vi "WORD report.vi"(7 "Report state":T1=enum."Close report", 8 "error in":errorcluster, 10 "Data in":variant) -> (0 "error out":errorcluster, 2 "Data out":variant)   [LabVIEW 2015, in "Report.lvlib"]
uses:
  Report.lvlib
  <vilib>/Utility/NIReport.llb/NI_report.lvclass
  <vilib>/Utility/NIReport.llb/Append Report Text (str wrap).vi
  <vilib>/Utility/NIReport.llb/NI_ReportGenerationCore.lvlib
  TypeDefs/Report data.ctl
  TypeDefs/Report state.ctl
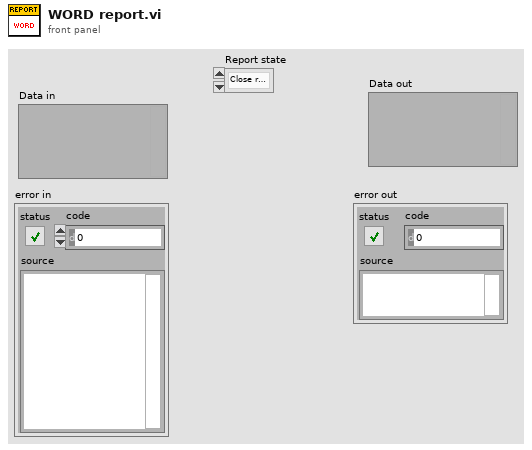
[diagram p1: front panel]
types:
  T1 = typedef "Report.lvlib/Report state.ctl" = enum16{"Create report", "Save data", "Save report", "Available printers", "Print report", "Close report"}
  T2 = enum16{"maximized", "minimized", "normal", "no change"}
  T3 = enum16{"Standard Report", "HTML", "Word", "Excel"}
  T4 = typedef "Report.lvlib/Report data.ctl" = cluster{"report ID":refnum<class "NI_report.lvclass">, "error":errorcluster}
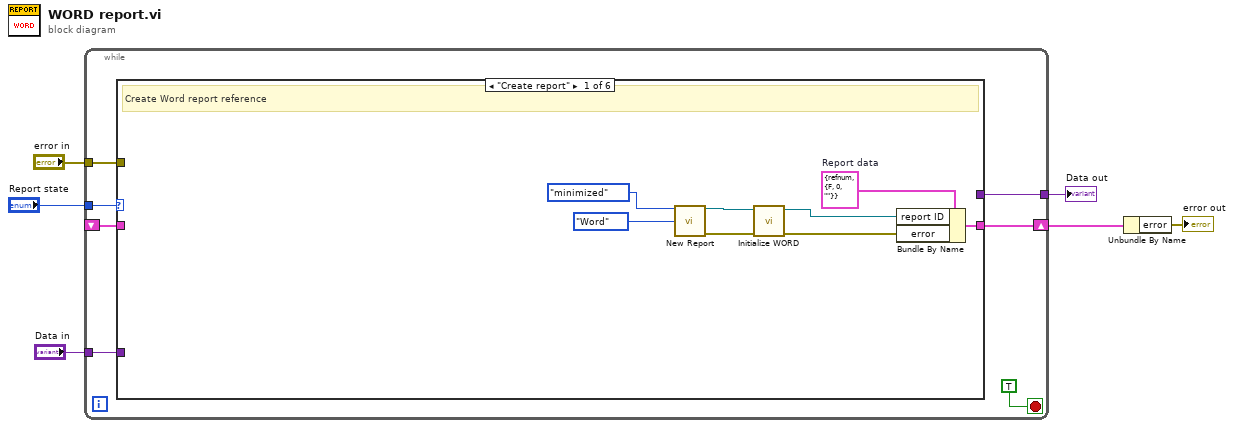
[diagram p0: block diagram]
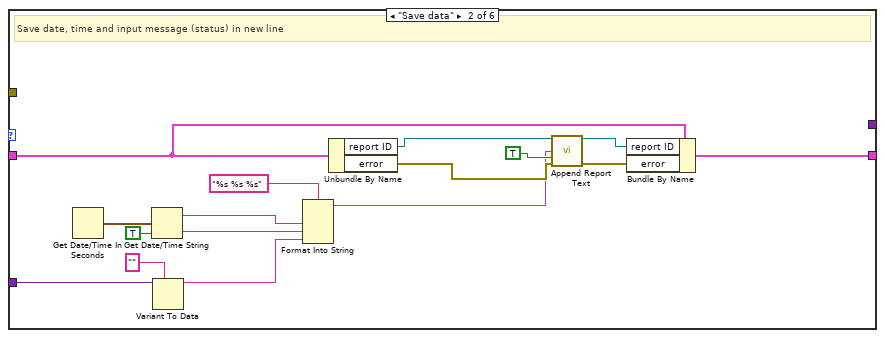
[diagram p2: hidden frame]
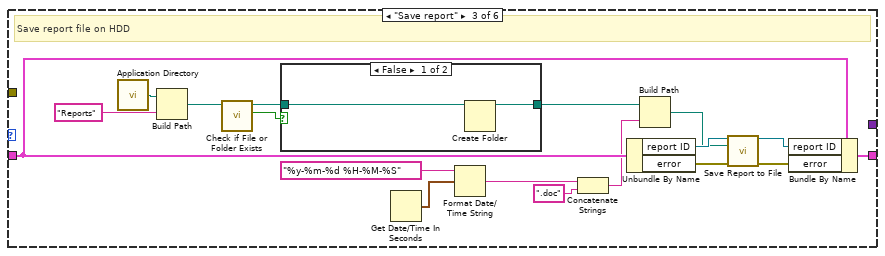
[diagram p3: hidden frame]
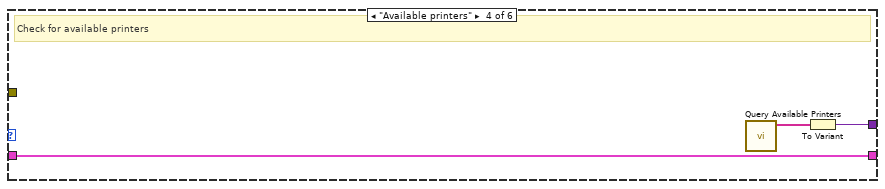
[diagram p5: hidden frame]
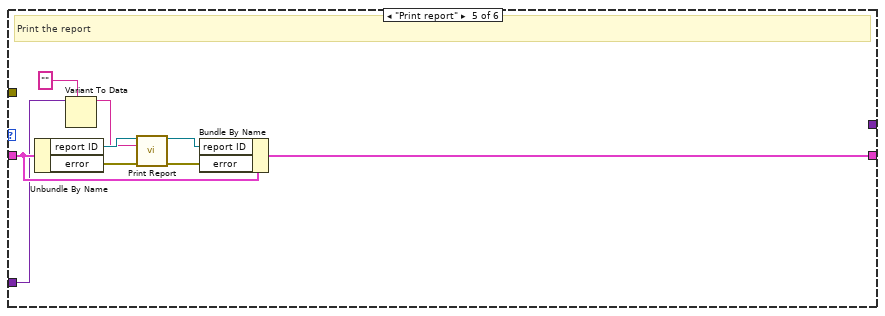
[diagram p6: hidden frame]
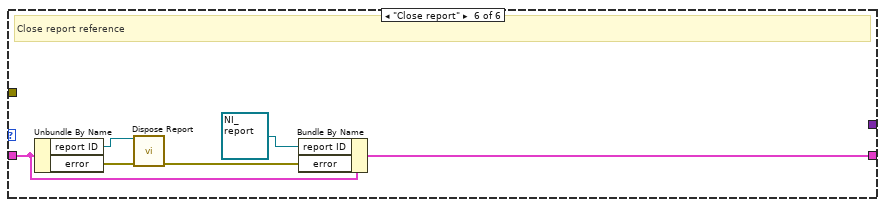
[diagram p7: hidden frame]
diagram:
  n1 = while {
    tunnel: "Report state" -> [w9]
    shift-right: [w11] -> w3
    shift-left: _ -> [w12]
    tunnel: "Data in" -> [w10]
    tunnel: "error in" -> [w8]
    tunnel: [w7] -> w1
    stop <- TRUE stop-if-true
    n2 = case shown="\"Create report\"" w9 {
      tunnel: w12 -> [_ w35 w55 w59 w68 w75]
      tunnel: [w21 w32 w54 w59 w67 w76] -> w11
      tunnel: w10 -> [_ w31 _ _ w64 _]
      tunnel: w8 -> [_ _ _ _ _ _]
      tunnel: [_ _ _ w60 _ _] -> w7
      frame "Create report" {
        w14 = T4 {"report ID"=refnum, "error"={"status"=FALSE, "code"=0, "source"=""}}  # Report data
        # "Create Word report reference"
        n3 = call <vilib>:"New Report.vi"("window state (normal)"=T2."minimized", "report type"=T3."Word") -> ("report out"=w18:refnum<class "NI_report.lvclass">, "error out"=w17:errorcluster)  [unwired: 12 in]
        n4 = call "Initialize WORD.vi"("error in (no error)"=w17, "NI_report in"=w18) -> ("error out"=w15:errorcluster, "NI_report out"=w16:refnum<class "NI_report.lvclass">)  [unwired: 8 in]
        n5 = Bundle By Name(cluster=w14, "report ID"=w16, "error"=w15) -> (w21:T4)
      }
      frame "Save data" {
        # "Save date, time and input message (status) in new line"
        n6 = Get Date/Time In Seconds() -> (seconds since 1Jan1904=w28:timestamp)
        n7 = Get Date/Time String(seconds (now)=w28, want seconds? (F)=TRUE) -> (date string=w26:string, time string=w25:string)  [unwired: 1 in]
        n8 = Variant To Data(type="", Variant=w31) -> (data=w24:string)  [unwired: 1 in, 1 out]
        n9 = Format Into String(format string="%s %s %s", w26, w25, w24) -> (resulting string=w22:string)  [unwired: 2 in, 1 out]
        n10 = Unbundle By Name(w35) -> ("report ID"=w37:refnum<class "NI_report.lvclass">, "error"=w36:errorcluster)
        n11 = call-poly <vilib>:"Append Report Text.vi"("report in"=w37, "text"=w22, "append on new line? (F)"=TRUE, "error in (no error)"=w36) -> ("report out"=w34:refnum<class "NI_report.lvclass">, "error out"=w33:errorcluster)  [unwired: 8 in, 2 out]
        n12 = Bundle By Name(cluster=w35, "report ID"=w34, "error"=w33) -> (w32:T4)
      }
      frame "Save report" {
        # "Save report file on HDD"
        n13 = call <vilib>:"Application Directory.vi"() -> ("Application Directory"=w43:path)
        n14 = Build Path(base path=w43, name or relative path="Reports") -> (appended path=w41:path)
        n15 = call <vilib>:"Check if File or Folder Exists.vi"("path"=w41) -> ("file or folder exists?"=w40:bool, "dup path"=w39:path)  [unwired: 8 in, 1 out]
        n16 = case shown="False" w40 {
          tunnel: w39 -> [w57 w58]
          tunnel: [w56 w58] -> w38
          frame False {
            n17 = Create Folder(path (use dialog)=w57) -> (created path=w56:path)  [unwired: 2 in, 2 out]
          }
          frame True {
          }
        }
        n18 = Get Date/Time In Seconds() -> (seconds since 1Jan1904=w48:timestamp)
        n19 = Format Date/Time String(time format string (%c)="%y-%m-%d %H-%M-%S", seconds (now)=w48) -> (date/time string=w46:string)  [unwired: 1 in]
        n20 = Concatenate Strings(w46, ".doc" ("string")) -> (w44:string)
        n21 = Unbundle By Name(w55) -> ("report ID"=w53:refnum<class "NI_report.lvclass">, "error"=w52:errorcluster)
        n22 = Build Path(base path=w38, name or relative path=w44) -> (appended path=w49:path)
        n23 = call-dynamic "Save Report to File.vi"("report in"=w53, "report file path"=w49, "error in (no error)"=w52) -> ("report out"=w51:refnum<class "NI_report.lvclass">, "error out"=w50:errorcluster)  [unwired: 11 in]
        n24 = Bundle By Name(cluster=w55, "report ID"=w51, "error"=w50) -> (w54:T4)
      }
      frame "Available printers" {
        # "Check for available printers"
        n25 = call <vilib>:"Query Available Printers.vi"() -> ("system configured printers"=w61:string[])  [unwired: 9 in, 2 out]
        n26 = To Variant(anything=w61) -> (Variant=w60:variant)
      }
      frame "Print report" {
        # "Print the report"
        n27 = Unbundle By Name(w68) -> ("report ID"=w70:refnum<class "NI_report.lvclass">, "error"=w69:errorcluster)
        n28 = Variant To Data(type="", Variant=w64) -> (data=w62:string)  [unwired: 1 in, 1 out]
        n29 = call-dynamic "Print Report.vi"("report in"=w70, "printer name (default)"=w62, "error in (no error)"=w69) -> ("report out"=w66:refnum<class "NI_report.lvclass">, "error out"=w65:errorcluster)  [unwired: 11 in]
        n30 = Bundle By Name(cluster=w68, "report ID"=w66, "error"=w65) -> (w67:T4)
      }
      frame "Close report" {
        # "Close report reference"
        n31 = Unbundle By Name(w75) -> ("report ID"=w74:refnum<class "NI_report.lvclass">, "error"=w73:errorcluster)
        n32 = call-dynamic "Dispose Report.vi"("report in"=w74, "error in (no error)"=w73) -> ("error out"=w71:errorcluster)  [unwired: 13 in]
        n33 = Bundle By Name(cluster=w75, "report ID"=refnum<class "NI_report.lvclass"> refnum, "error"=w71) -> (w76:T4)
      }
    }
  }
  "Data out" <- w1
  n34 = Unbundle By Name(w3) -> ("error"=→"error out":errorcluster)
